vi "GB2312 Encode.vi"(7 "个数":i32, 11 "字符串":string) -> (3 "数组":u8[](array[numeric]) format="%02x")   [LabVIEW 2016, in "DGUS.lvlib" / "DGUS.lvclass"]
uses:
  DGUS.lvclass
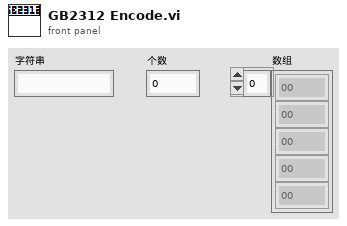
[diagram p1: front panel]
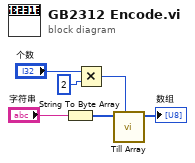
[diagram p0: block diagram]
diagram:
  n1 = String To Byte Array(string="字符串") -> (unsigned byte array=w5:u8[])
  n2 = Multiply(x="个数", y=2) -> (x*y=w2:i32)
  n3 = call "Till Array.vi"("字节个数"=w2, "input"=w5) -> ("output"=→"数组":u8[])  [unwired: 9 in]
